vi "Projection-Perspective.vi"(6 "Far Clipping Plane":sgl, 7 "Near Clipping Plane":sgl, 8 "error in (no error)":errorcluster, 9 "Aspect Ratio":sgl, 10 "Field of View":sgl, 11 "SceneGraphDisplay in":refnum<class "SceneGraphDisplay.lvclass">) -> (0 "error out":errorcluster, 3 "SceneGraphDisplay out":refnum<class "SceneGraphDisplay.lvclass">)   [LabVIEW 2015, in "SceneGraphDisplay.lvclass"]
doc: "Sets coordinates to render the scene in a frustum-shaped view, where you specify an angle for the horizontal and vertical viewing fields. This projection causes objects closer to the camera to appear larger in size. This method is similar to the Projection:Frustum method.\n\nQControl Class wrapper around the <b>SceneGraphDisplay : Projection:Perspective Method</b>.\n<b> </b> <b> </b>\n©2016 Q Software Innovations, LLC (QSI)\nwritten by Quentin Alldredge\nproduced in LabVIEW 2015\n\nsupport@qsoftwareinnovations.com\nwww.qsoftwareinnovations.com\n\nAll rights reserved.\n\nRedistribution and use in source and binary forms, with or without modification, are permitted provided that the following conditions are met:\n\n * Redistributions of source code must retain the above copyright notice, this list of conditions and the following disclaimer.\n * Redistributions in binary form must reproduce the above copyright notice, this list of conditions and the following disclaimer in the documentation and/or other materials provided with the distribution.\n * Neither the name of Q Software Innovations, LLC. nor the names of its contributors may be used to endorse or promote products derived from this software without specific prior written permission.\n\nTHIS SOFTWARE IS PROVIDED BY THE COPYRIGHT HOLDERS AND CONTRIBUTORS \"AS IS\" AND ANY EXPRESS OR IMPLIED WARRANTIES, INCLUDING, BUT NOT LIMITED TO, THE IMPLIED WARRANTIES OF MERCHANTABILITY AND FITNESS FOR A PARTICULAR PURPOSE ARE DISCLAIMED. IN NO EVENT SHALL THE COPYRIGHT OWNER OR CONTRIBUTORS BE LIABLE FOR ANY DIRECT, INDIRECT, INCIDENTAL, SPECIAL, EXEMPLARY, OR CONSEQUENTIAL DAMAGES (INCLUDING, BUT NOT LIMITED TO, PROCUREMENT OF SUBSTITUTE GOODS OR SERVICES; LOSS OF USE, DATA, OR PROFITS; OR BUSINESS INTERRUPTION) HOWEVER CAUSED AND ON ANY THEORY OF LIABILITY, WHETHER IN CONTRACT, STRICT LIABILITY, OR TORT (INCLUDING NEGLIGENCE OR OTHERWISE) ARISING IN ANY WAY OUT OF THE USE OF THIS SOFTWARE, EVEN IF ADVISED OF THE POSSIBILITY OF SUCH DAMAGE."
uses:
  SceneGraphDisplay.lvclass
  SceneGraphDisplay.lvclass/SceneGraphDisplay.ctl
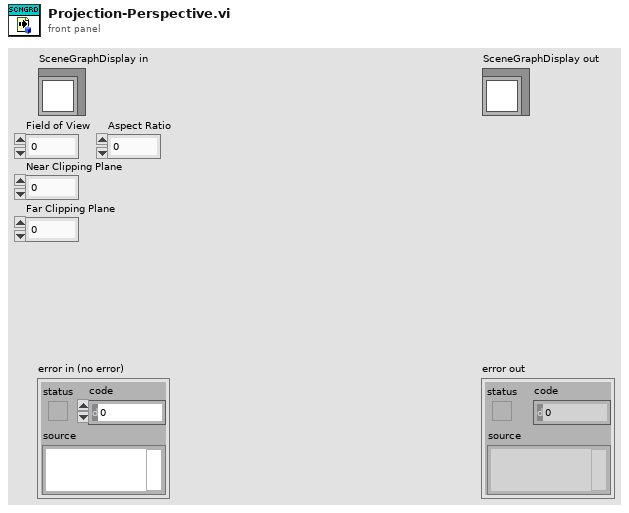
[diagram p1: front panel]
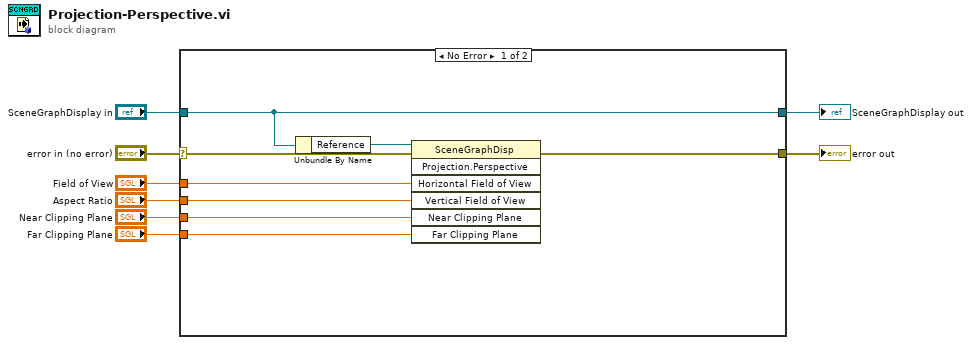
[diagram p0: block diagram]
diagram:
  n1 = case shown="No Error" "error in (no error)" {
    selector: "error in (no error)" -> [w16 w18]
    tunnel: [w15 w18] -> w7
    tunnel: [w14 w17] -> w5
    tunnel: "SceneGraphDisplay in" -> [w14 w17]
    tunnel: "Field of View" -> [w12 _]
    tunnel: "Aspect Ratio" -> [w11 _]
    tunnel: "Near Clipping Plane" -> [w10 _]
    tunnel: "Far Clipping Plane" -> [w9 _]
    frame No Error {
      n2 = Unbundle By Name(w14) -> ("Reference"=w13:refnum<vi>)
      n3 = invoke class="SceneGraphDisp" method="Projection.Perspective"(reference=w13, error in=w16, "Horizontal Field of View"=w12, "Vertical Field of View"=w11, "Near Clipping Plane"=w10, "Far Clipping Plane"=w9) -> (error out=w15:errorcluster)  [unwired: 1 in, 6 out]
    }
    frame Error {
    }
  }
  "error out" <- w7
  "SceneGraphDisplay out" <- w5
